vi "Dependency Generator.vi"() -> ()   [LabVIEW 2011, in "LMH-Toolbox.lvlib" / "LMH-Installer Tools.lvlib"]
uses:
  LMH-Installer Tools.lvlib
  Private/Type Defs/User Dependency.ctl
  <vilib>/Utility/file.llb/Write To Spreadsheet File (string).vi
  <vilib>/Utility/file.llb/Read From Spreadsheet File (string).vi
  LMH-Toolbox.lvlib
panel:
  out "Current Config":string
  in  "Save As Button":bool
  in  "Cancel Button":bool
  in  "Save Button":bool
  in  "Open Button":bool
  in  "Dependencies":T1[](array[typedef])
  # "Use this wizard to configure dependencies to be installed using\n JKI VI Package Manager and the LVH Dependency Installer."
  # "Name - \n\n\nVersion - \n\n\nTest VI Path - \n\n\n\n\n\nSource URL -\n\n\nInstaller Arguments -"
  # "The name of the dependency.  The will be visible to the  user during installation.\n\nThe version of the dependency. The will be visible to  the user during installation.\n\nA VI to run on the users system to test if the dependency is met.  The VI's connector pane must match the template and return true if the  dependency is met.\n\n The URL to download the dependency installer if necissary.\n\nCommand line arguments to pass to the installer.  This can be used to perform a quite install for example."
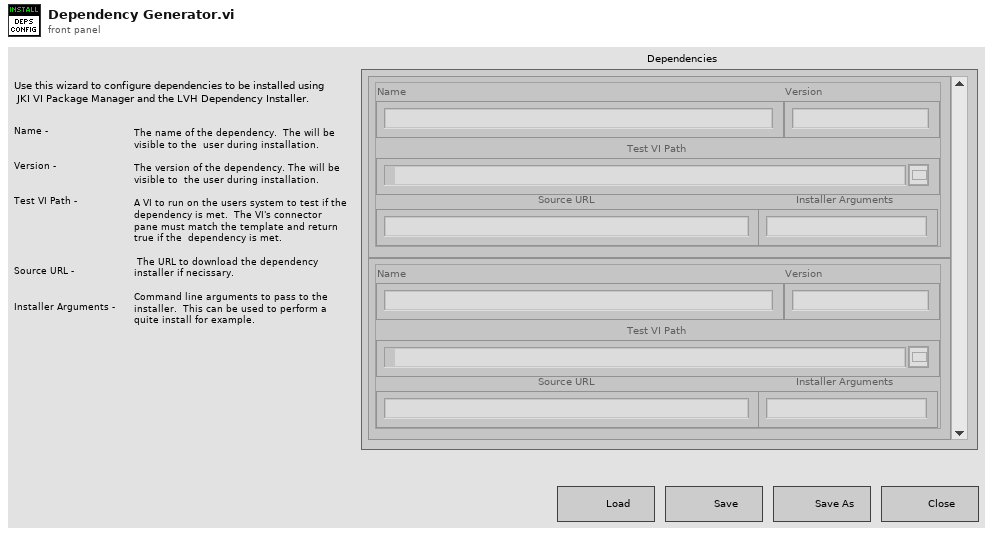
[diagram p1: front panel]
types:
  T1 = typedef "LMH-Toolbox.lvlib/LMH-Installer Tools.lvlib/User Dependency.ctl" = cluster{"Name":string, "Version":string, "Test VI Path":path, "Source URL":string, "Installer Arguments":string}
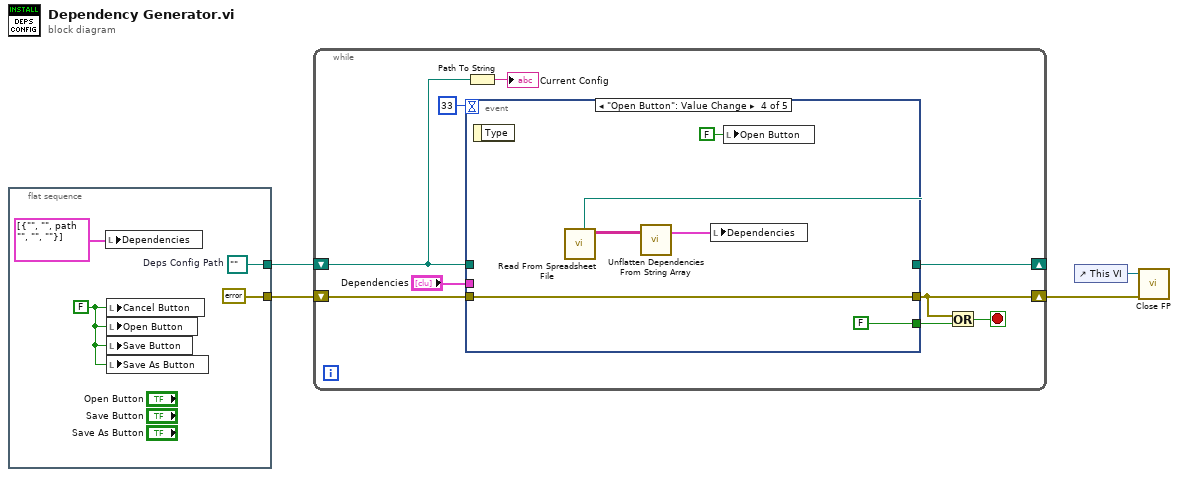
[diagram p0: block diagram]
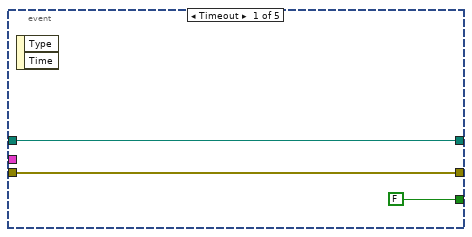
[diagram p2: hidden frame]
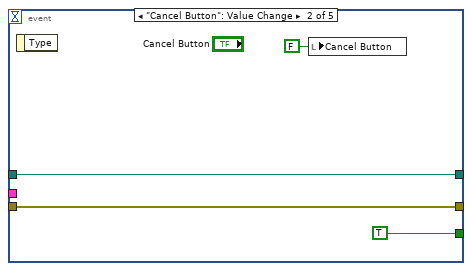
[diagram p3: hidden frame]
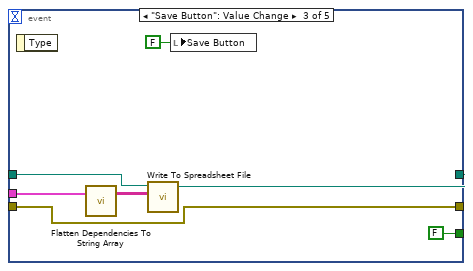
[diagram p4: hidden frame]
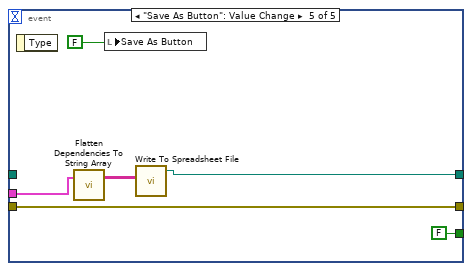
[diagram p5: hidden frame]
diagram:
  n1 = flat-sequence {
    tunnel: [errorcluster {"status"=FALSE, "code"=0, "source"=""} ("error constant")] -> w4
    tunnel: [w7] -> w3
    frame #0 {
      w6 = FALSE ("Cancel Button")
      w7 = path ""  # Deps Config Path
      n2 = local write "Dependencies"(T1[] [{"Name"="", "Version"="", "Test VI Path"=path "", "Source URL"="", "Installer Arguments"=""}] ("Dependecies")) -> ()
      n3 = local write "Cancel Button"(w6) -> ()
      n4 = local write "Open Button"(w6) -> ()
      n5 = local write "Save Button"(w6) -> ()
      n6 = local write "Save As Button"(w6) -> ()
    }
  }
  n7 = while {
    shift-right: [w11] -> _
    shift-left: w3 -> [w9]
    shift-right: [w13] -> w1
    shift-left: w4 -> [w16]
    stop <- w14 stop-if-true
    n8 = event shown="[3] \"Open Button\": Value Change" {
      selector: _ -> [_ _ _ _ _]
      dyn-events: _ -> [_ _ _ _ _]
      timeout: 33 -> [_ _ _ _ _]
      tunnel: [FALSE TRUE FALSE FALSE FALSE] -> w15
      tunnel: w16 -> [w19 w21 w25 w35 w42]
      tunnel: [w19 w21 w25 w35 w42] -> w13
      tunnel: "Dependencies" -> [_ _ w29 _ w40]
      tunnel: w9 -> [w18 w22 w27 _ _]
      tunnel: [w18 w22 w26 w36 w39] -> w11
      event Timeout {
        n9 = event-data() -> ()  [unwired: 1 in, 2 out]
      }
      event "Cancel Button": Value Change {
        n10 = event-data() -> ()  [unwired: 1 in, 1 out]
        n11 = local write "Cancel Button"(FALSE ("Cancel Button")) -> ()
      }
      event "Save Button": Value Change {
        n12 = event-data() -> ()  [unwired: 1 in, 1 out]
        n13 = call "Flatten Dependencies To String Array.vi"("User Deps"=w29) -> ("User Deps"=w28:string[][])  [unwired: 2 in]
        n14 = call-poly <vilib>:"Write To Spreadsheet File.vi"("2D data"=w28, "file path (dialog if empty)"=w27) -> ("new file path (Not A Path if cancelled)"=w26:path)  [unwired: 6 in]
        n15 = local write "Save Button"(FALSE ("Save Button")) -> ()
      }
      event "Open Button": Value Change {
        n16 = event-data() -> ()  [unwired: 1 in, 1 out]
        n17 = call-poly <vilib>:"Read From Spreadsheet File.vi"() -> ("all rows"=w34:string[][], "new file path (Not A Path if cancelled)"=w36:path)  [unwired: 7 in, 3 out]
        n18 = call "Unflatten Dependencies From String Array.vi"("Flattened Dependencies"=w34) -> ("User Deps"=w33:T1[])  [unwired: 1 in, 1 out]
        n19 = local write "Dependencies"(w33) -> ()
        n20 = local write "Open Button"(FALSE ("Open Button")) -> ()
      }
      event "Save As Button": Value Change {
        n21 = event-data() -> ()  [unwired: 1 in, 1 out]
        n22 = call "Flatten Dependencies To String Array.vi"("User Deps"=w40) -> ("User Deps"=w41:string[][])  [unwired: 2 in]
        n23 = local write "Save As Button"(FALSE ("Save As Button")) -> ()
        n24 = call-poly <vilib>:"Write To Spreadsheet File.vi"("2D data"=w41) -> ("new file path (Not A Path if cancelled)"=w39:path)  [unwired: 7 in]
      }
    }
    n25 = Path To String(path=w9) -> (string=→"Current Config":string)
    n26 = Or(x=w13, y=w15) -> (x .or. y?=w14:bool)
  }
  n27 = control-ref of="This VI"() -> (w2:refnum<vi>)
  n28 = call "Close FP.vi"("Error In"=w1, "VI Ref"=w2) -> ()  [unwired: 9 in, 1 out]
